vi "Initialize.vi"(8 "error in (no error)":errorcluster, 11 "DemoStage in":refnum<class "DemoStage.lvclass">) -> (0 "error out":errorcluster, 3 "DemoStage out":refnum<class "DemoStage.lvclass">)   [LabVIEW 2020, in "DemoStage.lvlib" / "DemoStage.lvclass"]
uses:
  DemoStage.lvclass
  Hardware Abstraction Layer/Component/Stage/Stage/Stage.lvclass
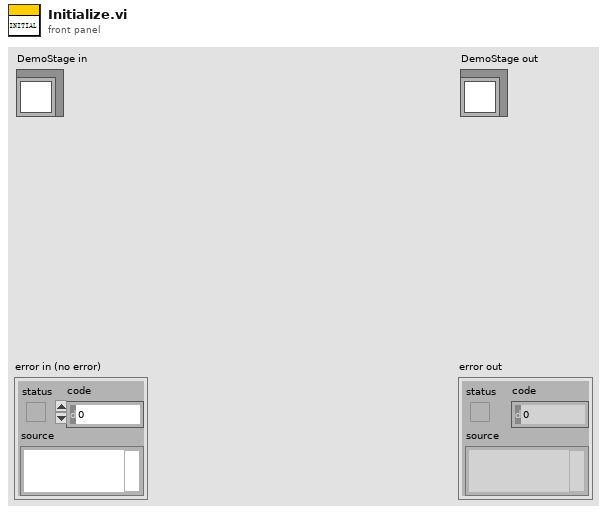
[diagram p1: front panel]
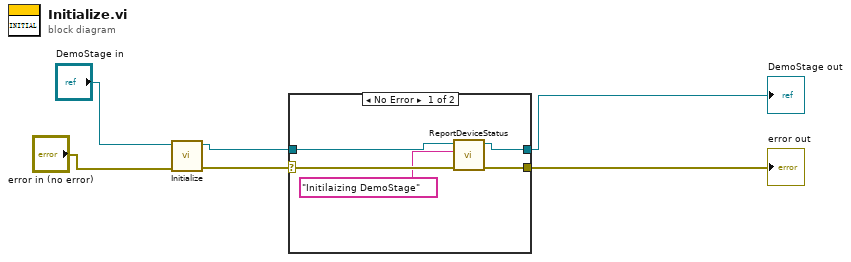
[diagram p0: block diagram]
diagram:
  n1 = call-parent "Initialize.vi"("error in (no error)"="error in (no error)", "Stage in"="DemoStage in") -> ("error out"=w3:errorcluster, "Stage out"=w4:refnum<class "DemoStage.lvclass">)  [unwired: 8 in]
  n2 = case shown="No Error" w3 {
    selector: w3 -> [w11 w13]
    tunnel: [w10 w13] -> w2
    tunnel: w4 -> [w9 w12]
    tunnel: [w8 w12] -> w1
    frame No Error {
      n3 = call-dynamic "ReportDeviceStatus.vi"("error in (no error)"=w11, "Status"="Initilaizing DemoStage", "Device in"=w9) -> ("error out"=w10:errorcluster, "Device out"=w8:refnum<class "DemoStage.lvclass">)  [unwired: 7 in]
    }
    frame Error {
    }
  }
  "error out" <- w2
  "DemoStage out" <- w1
